vi "Get Exotic Types for Tests.vi"() -> (3 "exotic types":variant[](array[variant]))   [LabVIEW 2020]
panel:
  in  "Waveform":waveform(dbl)={"t0"=timestamp(0 s since 1904-01-01), "dt"=0.0, "Y"=[]}
  in  "IMAQ Session":refnum<k11>
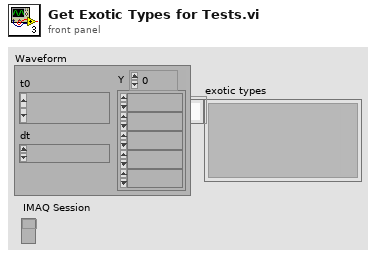
[diagram p1: front panel]
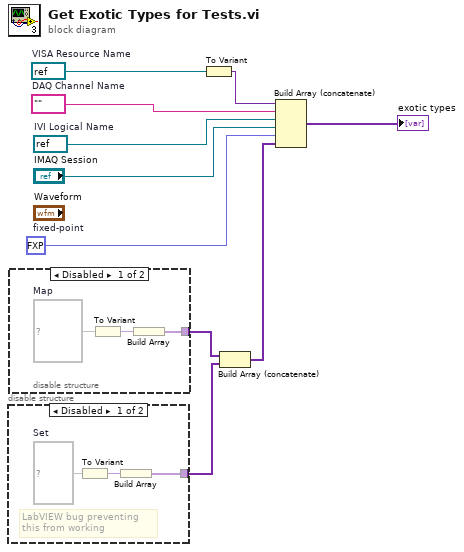
[diagram p0: block diagram]
diagram:
  w5 = fxp<+/-,32,16> 0.0  # fixed-point
  w7 = refnum<k15> refnum  # IVI Logical Name
  w8 = tag ""  # DAQ Channel Name
  w10 = refnum<visa-resource-name> refnum  # VISA Resource Name
  n1 = disable-structure shown="Disabled" {
    disable-tunnel: [w12 _] -> w2
    frame Disabled {
      w13 = set{string} {}  # Set
      # "LabVIEW bug preventing this from working"
      n2 = To Variant(anything=w13) -> (Variant=w11:variant)
      n3 = Build Array(w11) -> (w12:variant[])
    }
    frame Enabled {
    }
  }
  n4 = disable-structure shown="Disabled" {
    disable-tunnel: [w14 _] -> w1
    frame Disabled {
      w16 = map{string, i32} {}  # Map
      n5 = To Variant(anything=w16) -> (Variant=w15:variant)
      n6 = Build Array(w15) -> (w14:variant[])
    }
    frame Enabled {
    }
  }
  n7 = To Variant(anything=w10) -> (Variant=w9:variant)
  n8 = Build Array (concatenate)(w1, w2) -> (w4:variant[])
  n9 = Build Array (concatenate)(w9, w8, w7, "IMAQ Session", w5, w4) -> (→"exotic types":variant[])
